vi "RecordWrite.vi"(1 "Array":dbl[](array[numeric]), 2 "start time":u32, 3 "refnum in":refnum<file>) -> (0 "ref file":refnum<file>)   [LabVIEW 2015]
panel:
  out "error out":errorcluster
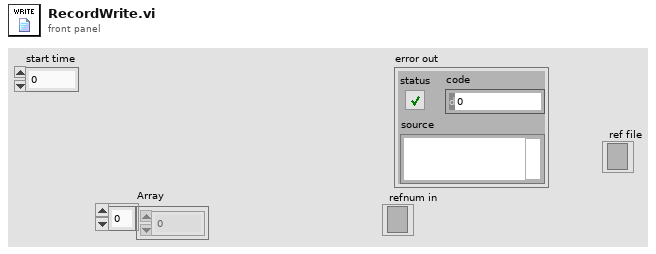
[diagram p1: front panel]
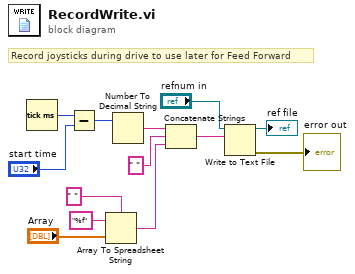
[diagram p0: block diagram]
diagram:
  # "Record joysticks during drive to use later for Feed Forward"
  n1 = Tick Count (ms)() -> (millisecond timer value=w4:u32)
  n2 = Subtract(x=w4, y="start time") -> (x-y=w8:u32)
  n3 = Array To Spreadsheet String(delimiter (Tab)=" ", array="Array", 3:"%f" ("format string")) -> (spreadsheet string=w10:string)
  n4 = Number To Decimal String(number=w8) -> (decimal integer string=w7:string)  [unwired: 1 in]
  n5 = Concatenate Strings(w7, " " ("string"), w10) -> (w6:string)
  n6 = Write to Text File(file (use dialog)="refnum in", text=w6) -> (refnum out=→"ref file":refnum<file>, error out=→"error out":errorcluster)  [unwired: 2 in, 1 out]
